vi "Set Channel Default State.vi"(8 "error in (no error)":errorcluster, 10 "State":string, 11 "Channel Ref in":T1 format="%.0x") -> (0 "error out":errorcluster, 3 "Channel Ref out":T1=18446744073709551615 format="%.0x")   [LabVIEW 2017, in "SLSC Switch Scripting.lvlib"]
uses:
  SLSC Switch Scripting.lvlib
  <vilib>/NI Veristand/Custom Device API/Custom Device Item Ref.ctl
  <vilib>/NI VeriStand/Custom Device API/Custom Device API.lvlib
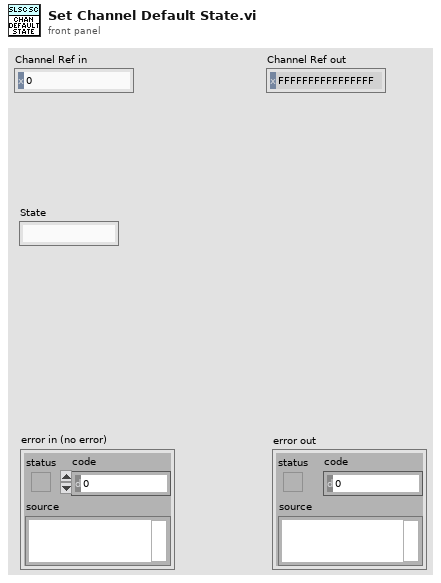
[diagram p1: front panel]
types:
  T1 = typedef "Custom Device API.lvlib/Custom Device Item Ref.ctl" = u64
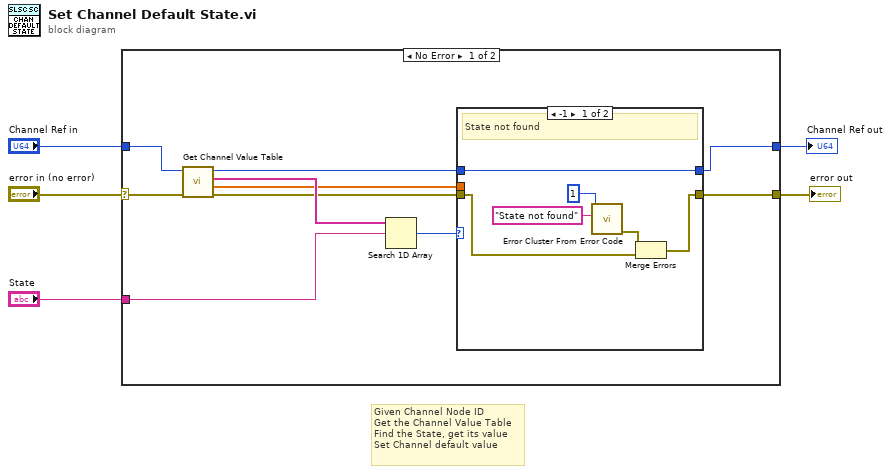
[diagram p0: block diagram]
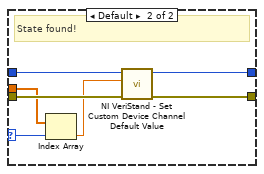
[diagram p2: hidden frame]
diagram:
  # "Given Channel Node ID\nGet the Channel Value Table\nFind the State, get its value\nSet Channel default value"
  n1 = case shown="No Error" "error in (no error)" {
    selector: "error in (no error)" -> [w14 w30]
    tunnel: [w6 w30] -> w1
    tunnel: "Channel Ref in" -> [w15 w29]
    tunnel: [w7 w29] -> w3
    tunnel: "State" -> [w12 _]
    frame No Error {
      n2 = call "Get Channel Value Table.vi"("error in (no error)"=w14, "Channel Ref in"=w15) -> ("error out"=w10:errorcluster, "Values"=w9:dbl[], "States"=w13:string[], "Channel Ref out"=w11:T1)  [unwired: 6 in]
      n3 = Search 1D Array(1D array=w13, element=w12) -> (index of element=w8:i32)  [unwired: 1 in]
      n4 = case shown="-1" w8 {
        selector: w8 -> [_ w24]
        tunnel: w11 -> [w19 w28]
        tunnel: w10 -> [w17 w27]
        tunnel: w9 -> [_ w26]
        tunnel: [w19 w23] -> w7
        tunnel: [w16 w22] -> w6
        frame -1 {
          # "State not found"
          n5 = call <vilib>:"Error Cluster From Error Code.vi"("error message (\"\")"="State not found" ("error message (\"\")"), "error code (0)"=1) -> ("error out"=w18:errorcluster)  [unwired: 7 in]
          n6 = Merge Errors(w18, w17) -> (w16:errorcluster)
        }
        frame Default {
          # "State found!"
          n7 = Index Array(array=w26, index=w24) -> (element=w25:dbl)
          n8 = call <vilib>:"NI VeriStand - Set Custom Device Channel Default Value.vi"("error in (no error)"=w27, "Default Value"=w25, "Channel Ref in"=w28) -> ("error out"=w22:errorcluster, "Channel Ref out"=w23:T1)  [unwired: 7 in]
        }
      }
    }
    frame Error {
    }
  }
  "Channel Ref out" <- w3
  "error out" <- w1
